vi "Paths okay.vi"(11 "Paths":T1) -> (2 "passed":bool, 3 "Paths out":T1)   [LabVIEW 2012]
uses:
  Paths.ctl
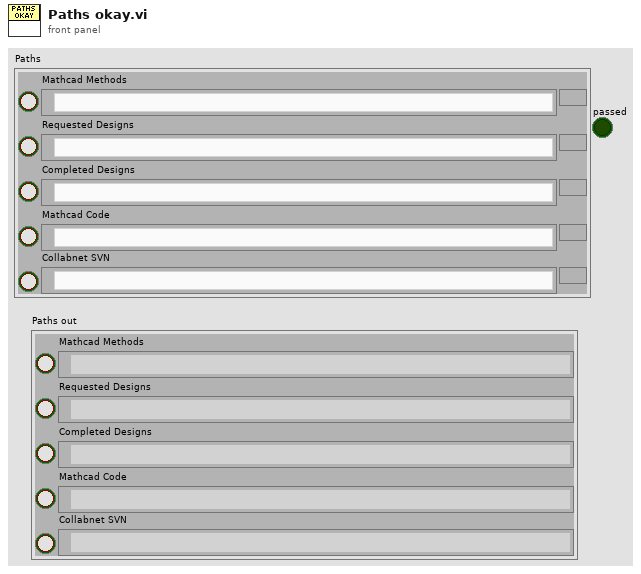
[diagram p1: front panel]
types:
  T1 = typedef "Paths.ctl" = cluster{"Mathcad Methods":path, "Requested Designs":path, "Completed Designs":path, "Mathcad Code":path, "Collabnet SVN":path, "Mathcad Methods ok":bool, "Requested Designs ok":bool, "Completed Designs ok":bool, "Mathcad Code ok":bool, "Collabnet SVN":bool}
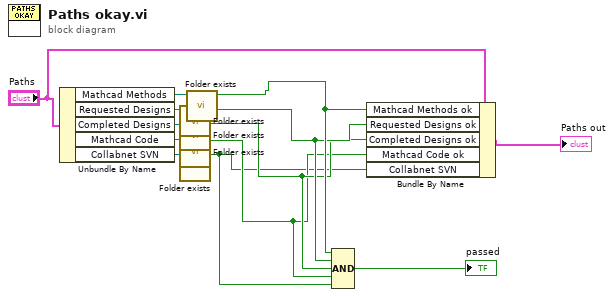
[diagram p0: block diagram]
diagram:
  n1 = Unbundle By Name("Paths") -> ("Mathcad Methods"=w8:path, "Requested Designs"=w11:path, "Completed Designs"=w10:path, "Mathcad Code"=w9:path, "Collabnet SVN"=w3:path)
  n2 = call "Folder exists.vi"("path"=w11) -> ("folder exists?"=w6:bool)  [unwired: 10 in]
  n3 = call "Folder exists.vi"("path"=w10) -> ("folder exists?"=w5:bool)  [unwired: 10 in]
  n4 = call "Folder exists.vi"("path"=w9) -> ("folder exists?"=w4:bool)  [unwired: 10 in]
  n5 = call "Folder exists.vi"("path"=w3) -> ("folder exists?"=w2:bool)  [unwired: 10 in]
  n6 = call "Folder exists.vi"("path"=w8) -> ("folder exists?"=w7:bool)  [unwired: 10 in]
  n7 = Compound Arithmetic op=AND(w7, w6, w5, w4, w2) -> (→"passed":bool)
  n8 = Bundle By Name(cluster="Paths", "Mathcad Methods ok"=w7, "Requested Designs ok"=w6, "Completed Designs ok"=w5, "Mathcad Code ok"=w4, "Collabnet SVN"=w2) -> (→"Paths out":T1)
